vi "Sub_square_from_csv.vi"(11 "To Flatten":dbl[][](array[numeric])) -> (3 "Square":dbl[][](array[numeric]))   [LabVIEW 2021]
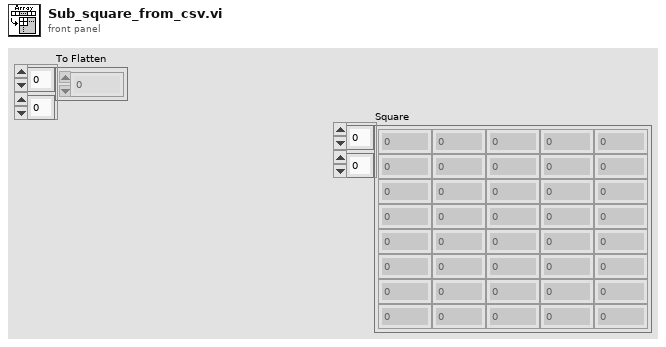
[diagram p1: front panel]
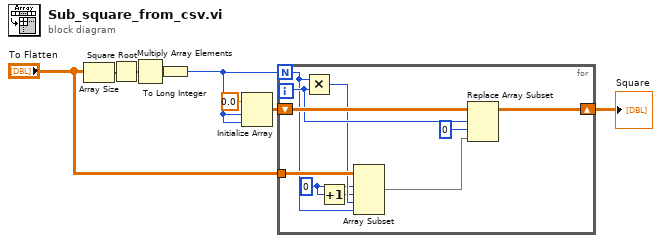
[diagram p0: block diagram]
diagram:
  n1 = Array Size(array="To Flatten") -> (size(s)=w5:i32[])
  n2 = Square Root(x=w5) -> (sqrt(x)=w8:dbl[])
  n3 = Multiply Array Elements(1:w8) -> (0:w7:dbl)
  n4 = To Long Integer(number=w7) -> (32bit integer=w4:i32)
  n5 = Initialize Array(0.0 ("element"), w4, w4) -> (w2:dbl[][])
  n6 = for {
    N: w4 -> [w13]
    tunnel: "To Flatten" -> [w16]
    shift-right: [w17] -> w1
    shift-left: w2 -> [w18]
    i -> [w15]
    w12 = 0 ("index")
    n7 = Multiply(x=w13, y=w15) -> (x*y=w14:i32)
    n8 = Increment(x=w12) -> (x+1=w11:i32)
    n9 = Array Subset(array=w16, index (row)=w12, length (row)=w11, index (col)=w14, length (col)=w13) -> (w10:dbl[][])
    n10 = Replace Array Subset(array=w18, new element=w10, index (row)=w15, index (col)=0 ("disabled index (col)")) -> (w17:dbl[][])
  }
  "Square" <- w1
